vi "MB Ethernet Receive.vi"(7 "Slave":bool, 8 "error in (no error)":errorcluster, 10 "Transaction ID WR":u16, 11 "TCP in":refnum<class "TCP.lvclass">) -> (0 "error out":errorcluster, 1 "Exception Code":u8 format="%.0x", 2 "Modbus Data Unit":T2={"function"=1, "Data"=[]} {"function" items=["Read Discrete Inputs"=2, "Read Coils"=1, "Write Single Coil"=5, "Write Multiple Coils"=15, "Read Input Register"=4, "Read Holding Registers"=3, "Write Single Register"=6, "Write Multiple Registers"=16, "Read/Write Multiple Registers"=23, "Mask Write Register"=22, "Read FIFO Queue"=24, "Read File Record"=20, "Write File Record"=21, "Read Exception Status"=7, "Diagnostic"=8, "Get Com Event Counter"=11, "Get Com Event Log"=12, "Report Slave ID"=17, "Read Device Identification"=43]; "Data" format="%.0x"}, 3 "TCP out":refnum<class "TCP.lvclass">, 5 "MBAP Header":T1)   [LabVIEW 2019, in "NI_modbus_upd.lvlib"]
uses:
  Ctl/MB Modbus Data Unit.ctl
  Modbus Data Unit (PDU)/Function.ctl
  TCP/TCP.lvclass
  TCP/TCP.lvclass/TCP.ctl
  NI_modbus_upd.lvlib
panel:
  # "VI Name: MB Ethernet Receive.vi\nPurpose: Reads a Modbus message over Ethernet.\nReentrant VI, because its caller is also reentrant."
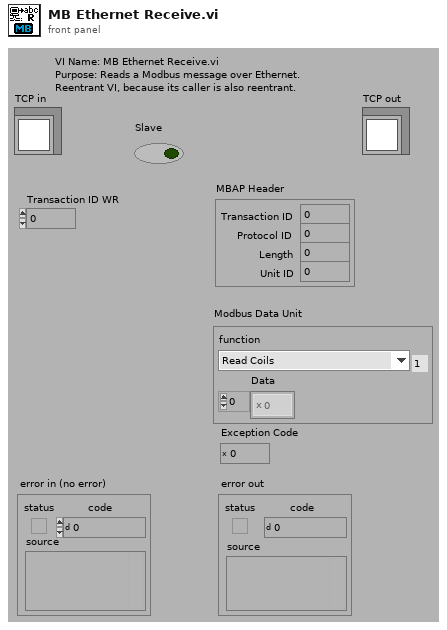
[diagram p1: front panel]
types:
  T1 = cluster{"Transaction ID":u16, "Protocol ID":u16, "Length":u16, "Unit ID":u8}
  T2 = typedef "NI_modbus_upd.lvlib/MB Modbus Data Unit.ctl" = cluster{"function":T3, "Data":u8[]}
  T3 = typedef "NI_modbus_upd.lvlib/Function.ctl" = u8
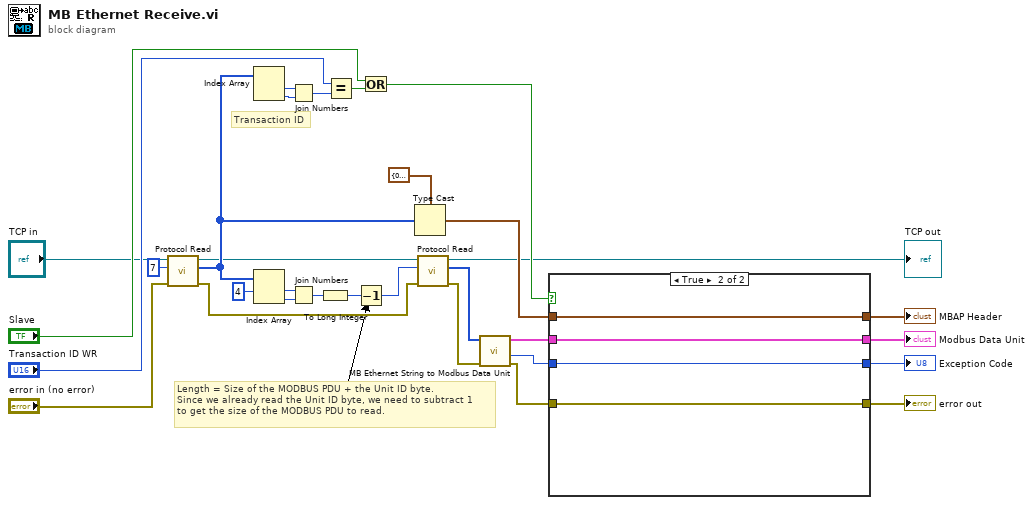
[diagram p0: block diagram]
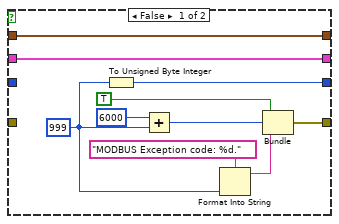
[diagram p2: hidden frame]
diagram:
  # "Length = Size of the MODBUS PDU + the Unit ID byte.\nSince we already read the Unit ID byte, we need to subtract 1\nto get the size of the MODBUS PDU to read."
  # "Transaction ID"
  n1 = call "Protocol Read.vi"("error in (no error)"="error in (no error)", "bytes to read"=7, "TCP in"="TCP in") -> ("error out"=w4:errorcluster, "data"=w8:u8[], "TCP out"=w6:refnum<class "TCP.lvclass">)  [unwired: 5 in, 1 out]
  n2 = Index Array(array=w8) -> (element #1=w30:u8, element #2=w31:u8)  [unwired: 2 in]
  n3 = Index Array(array=w8, index #1=4 ("index")) -> (element #1=w17:u8, element #2=w18:u8)  [unwired: 1 in]
  n4 = Join Numbers(hi=w30, lo=w31) -> ((hi.lo)=w12:u16)
  n5 = Join Numbers(hi=w17, lo=w18) -> ((hi.lo)=w20:u16)
  n6 = To Long Integer(number=w20) -> (32bit integer=w19:i32)
  n7 = Equal?(x="Transaction ID WR", y=w12) -> (x = y?=w14:bool)
  n8 = Decrement(x=w19) -> (x-1=w5:i32)
  n9 = Or(x="Slave", y=w14) -> (x .or. y?=w15:bool)
  n10 = Type Cast(type=T1 {"Transaction ID"=0, "Protocol ID"=0, "Length"=0, "Unit ID"=0} ("MBAP Header"), x=w8) -> (*(type *) &x=w28:T1)
  n11 = call "Protocol Read.vi"("error in (no error)"=w4, "bytes to read"=w5, "TCP in"=w6) -> ("error out"=w2:errorcluster, "data"=w1:u8[], "TCP out"=→"TCP out":refnum<class "TCP.lvclass">)  [unwired: 5 in, 1 out]
  n12 = call "MB Ethernet String to Modbus Data Unit.vi"("error in (no error)"=w2, "data"=w1) -> ("error out"=w26:errorcluster, "Exception Code"=w27:u8, "Modbus Data Unit"=w29:T2)  [unwired: 7 in]
  n13 = case shown="True" w15 {
    tunnel: [w32 w44] -> w25
    tunnel: [w34 w43] -> w23
    tunnel: [w36 w42] -> w22
    tunnel: [w33 w45] -> w24
    tunnel: w29 -> [w33 w45]
    tunnel: w28 -> [w32 w44]
    tunnel: w27 -> [_ w43]
    tunnel: w26 -> [_ w42]
    frame False {
      w35 = 999 ("32bit integer")
      n14 = To Unsigned Byte Integer(number=w35) -> (unsigned 8bit integer=w34:u8)
      n15 = Add(x=6000 ("New Error Code"), y=w35) -> (x+y=w39:i32)
      n16 = Format Into String(format string="MODBUS Exception code: %d.", w35) -> (resulting string=w41:string)  [unwired: 2 in, 1 out]
      n17 = Bundle(TRUE, w39, w41) -> (w36:errorcluster)  [unwired: 1 in]
    }
    frame True {
    }
  }
  "Exception Code" <- w23
  "Modbus Data Unit" <- w24
  "error out" <- w22
  "MBAP Header" <- w25
